vi "findCityv4.vi"(1 "limit":u16=10, 2 "API-key":string="1f08b39fd7a0b3e8daca028d6713f0316ab1cd82830e7bb362f85995e22aba7a", 3 "longitude":dbl=25.4651, 4 "latitude":dbl=65.0121, 6 "range":u16=10000) -> (0 "value":T1, 5 "not-found":bool)   [LabVIEW 2024]
uses:
  <vilib>/httpClient/LabVIEWHTTPClient.lvlib
panel:
  out "resulting string":string
  out "headers":string
  out "body":string
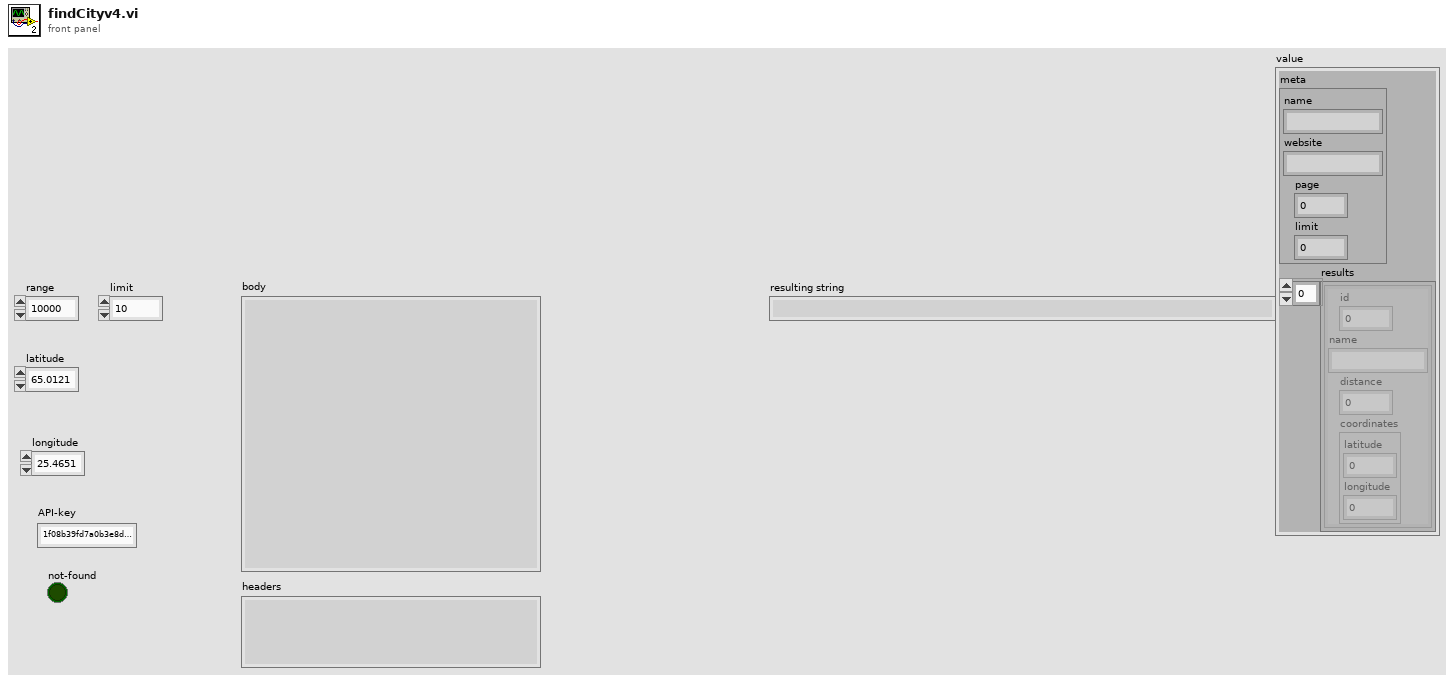
[diagram p1: front panel]
types:
  T1 = cluster{"meta":cluster{"name":string, "website":string, "page":dbl, "limit":dbl}, "results":cluster{"id":i32, "name":string, "distance":dbl, "coordinates":cluster{"latitude":dbl, "longitude":dbl}}[]}
  T2 = typedef "LabVIEWHTTPClient.lvlib/ClientHandle.ctl" = refnum<k1>
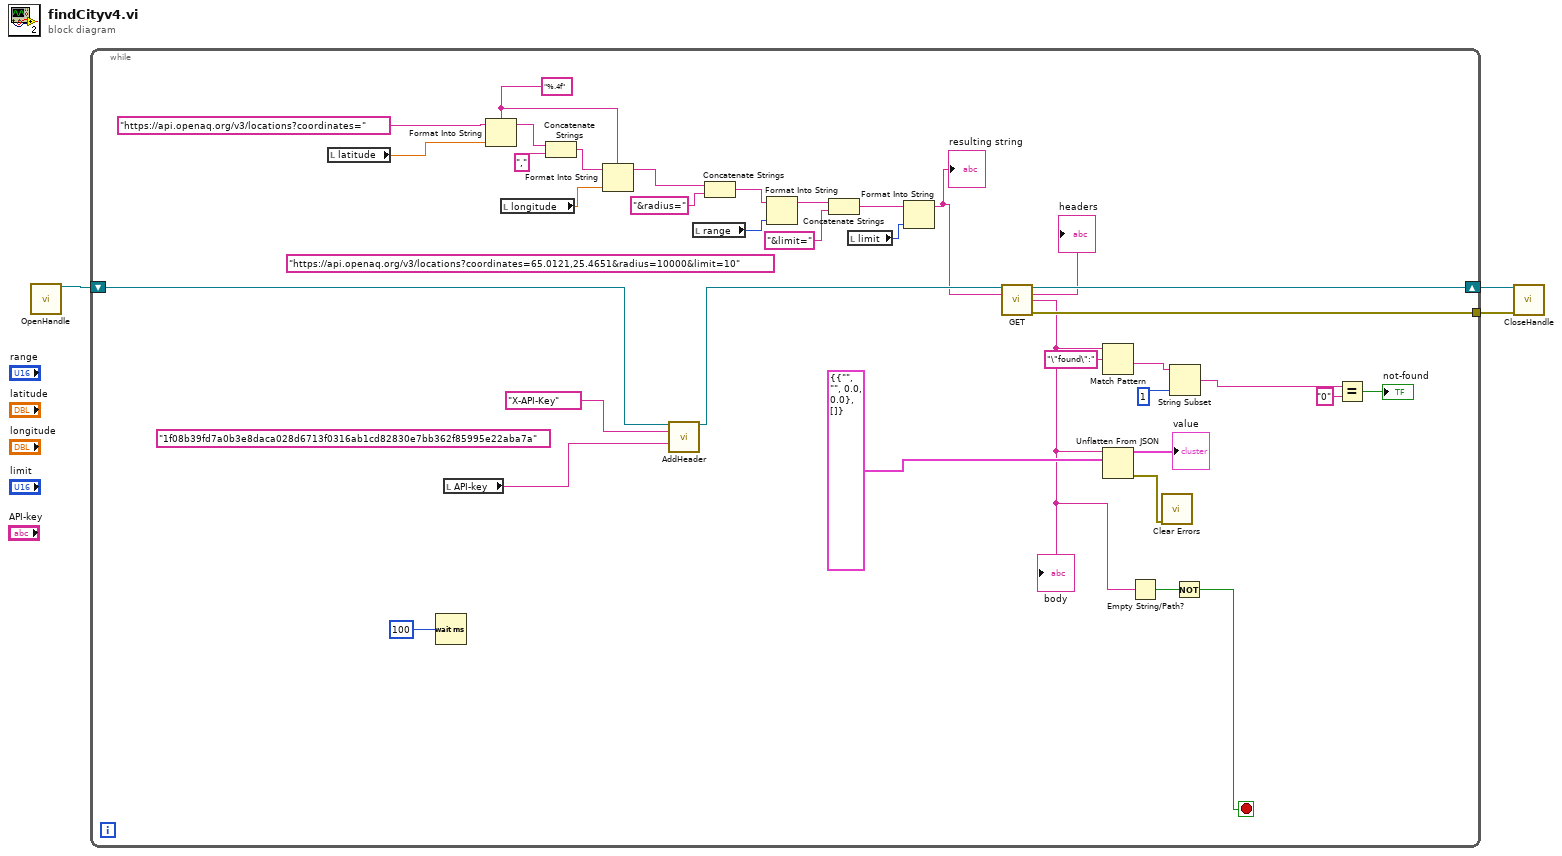
[diagram p0: block diagram]
diagram:
  n1 = call <vilib>:"OpenHandle.vi"() -> ("client handle out"=w1:T2)  [unwired: 14 in, 1 out]
  n2 = while {
    tunnel: [w38] -> w2
    shift-right: [w39] -> w3
    shift-left: w1 -> [w33]
    stop <- w30 stop-if-true
    w23 = "%.4f" ("format string")
    (unwired) "1f08b39fd7a0b3e8daca028d6713f0316ab1cd82830e7bb362f85995e22aba7a" ("value")
    (unwired) "https://api.openaq.org/v3/locations?coordinates=65.0121,25.4651&radius=10000&limit=10" ("url")
    n3 = local read "latitude"() -> (w29:dbl)
    n4 = Wait (ms)(milliseconds to wait=u32 100) -> ()  [unwired: 1 out]
    n5 = local read "API-key"() -> (w13:string)
    n6 = Format Into String(format string=w23, initial string="https://api.openaq.org/v3/locations?coordinates=" ("url"), w29) -> (resulting string=w27:string)  [unwired: 1 in, 1 out]
    n7 = local read "longitude"() -> (w24:dbl)
    n8 = Concatenate Strings(w27, "," ("string")) -> (w25:string)
    n9 = Format Into String(format string=w23, initial string=w25, w24) -> (resulting string=w22:string)  [unwired: 1 in, 1 out]
    n10 = call <vilib>:"AddHeader.vi"("client handle"=w33, "header"="X-API-Key", "value"=w13) -> ("client handle out"=w36:T2)  [unwired: 11 in, 1 out]
    n11 = local read "range"() -> (w19:u16)
    n12 = Concatenate Strings(w22, "&radius=" ("string")) -> (w20:string)
    n13 = Format Into String(initial string=w20, w19) -> (resulting string=w18:string)  [unwired: 2 in, 1 out]
    n14 = Concatenate Strings(w18, "&limit=" ("string")) -> (w16:string)
    n15 = local read "limit"() -> (w15:u16)
    n16 = Format Into String(initial string=w16, w15) -> (resulting string=w14:string)  [unwired: 2 in, 1 out]
    "resulting string" <- w14
    n17 = call <vilib>:"GET.vi"("client handle"=w36, "url"=w14) -> ("client handle out"=w39:T2, "headers"=→"headers":string, "body"=w11:string, "error out"=w38:errorcluster)  [unwired: 10 in]
    "body" <- w11
    n18 = Match Pattern(string=w11, regular expression="\"found\":") -> (after substring=w9:string)  [unwired: 1 in, 3 out]
    n19 = Unflatten From JSON(JSON string=w11, type and defaults=T1 {"meta"={"name"="", "website"="", "page"=0.0, "limit"=0.0}, "results"=[]}) -> (value=→"value":T1, error out=w12:errorcluster)  [unwired: 5 in]
    n20 = Empty String/Path?(string/path=w11) -> (empty?=w31:bool)
    n21 = call <vilib>:"Clear Errors.vi"("error in (no error)"=w12) -> ()  [unwired: 5 in, 2 out]
    n22 = String Subset(string=w9, length (rest)=1 ("length (rest)")) -> (substring=w7:string)  [unwired: 1 in]
    n23 = Not(x=w31) -> (.not. x?=w30:bool)
    n24 = Equal?(x=w7, y="0") -> (x = y?=→"not-found":bool)
  }
  n25 = call <vilib>:"CloseHandle.vi"("client handle"=w3, "error in (no error)"=w2) -> ()  [unwired: 13 in, 1 out]
